vi "FlatToRichnixnet_grpc_SetPropertyRequest.vi"(5 "OutputClusterType":T1, 11 "InputCluster":T3) -> (3 "OutputCluster":T1)   [LabVIEW 2025, in "grpc-xnet_client.lvlib"]
uses:
  nixnet_grpc_SetPropertyRequest_Flat.ctl
  nidevice_grpc_Session_Flat.ctl
  nixnet_grpc_Property.ctl
  nixnet_grpc_U32Array_Flat.ctl
  nixnet_grpc_DbRefArray_Flat.ctl
  nixnet_grpc_EptRxFilterArray_Flat.ctl
  nixnet_grpc_EptRxFilter_Flat.ctl
  nixnet_grpc_SetPropertyRequest.ctl
  nixnet_grpc_SetPropertyRequest_property_id_enum/nixnet_grpc_SetPropertyRequest_property_id_enum.lvclass
  nixnet_grpc_SetPropertyRequest_property_value/nixnet_grpc_SetPropertyRequest_property_value.lvclass
  nidevice_grpc_Session.ctl
  grpc-xnet_client.lvlib
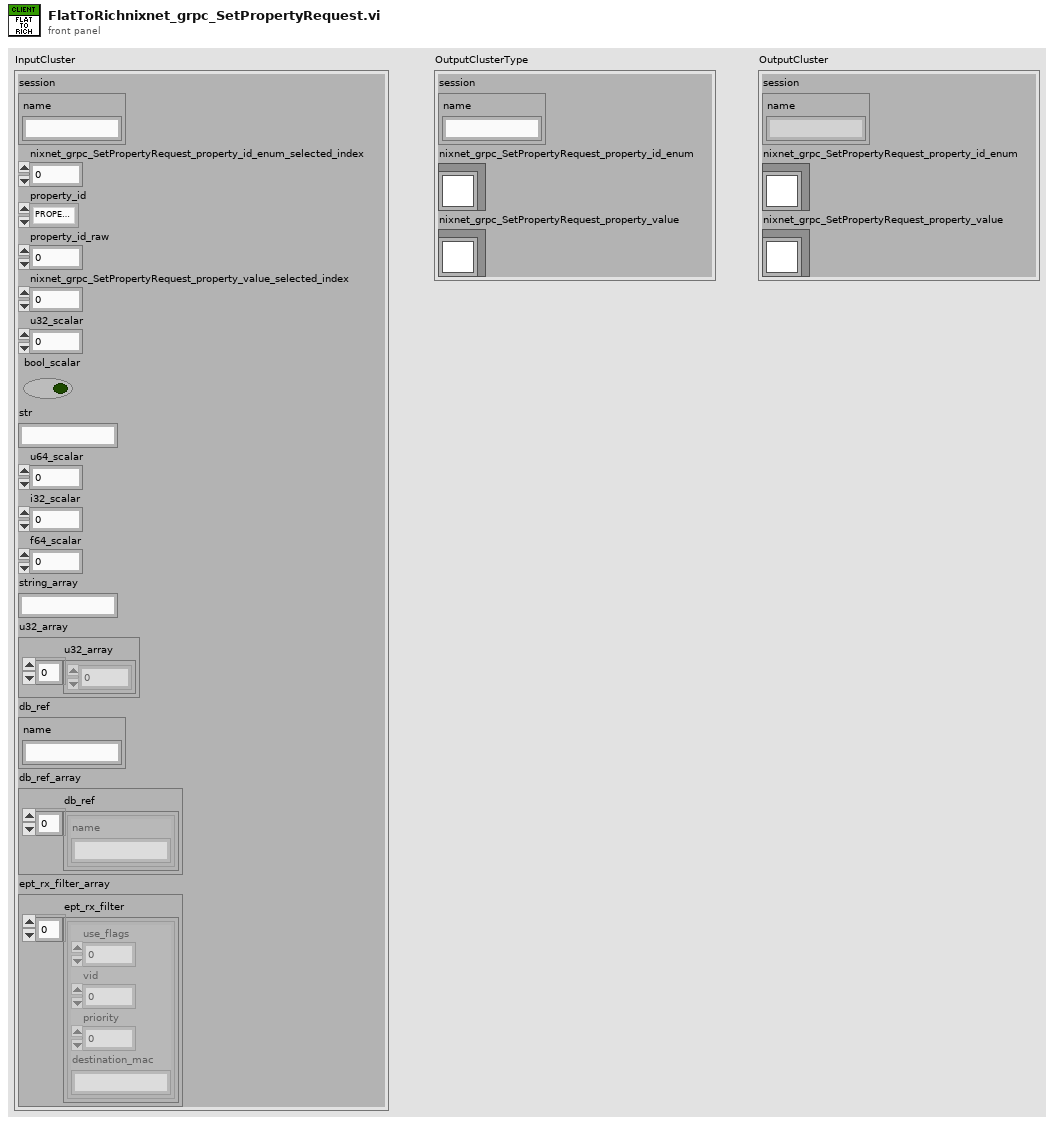
[diagram p1: front panel]
types:
  T1 = typedef "grpc-xnet_client.lvlib/nixnet_grpc_SetPropertyRequest.ctl" = cluster{"session":T2, "nixnet_grpc_SetPropertyRequest_property_id_enum":refnum<class "nixnet_grpc_SetPropertyRequest_property_id_enum.lvclass">, "nixnet_grpc_SetPropertyRequest_property_value":refnum<class "nixnet_grpc_SetPropertyRequest_property_value.lvclass">}
  T2 = typedef "grpc-xnet_client.lvlib/nidevice_grpc_Session.ctl" = cluster{"name":string}
  T3 = typedef "grpc-xnet_client.lvlib/nixnet_grpc_SetPropertyRequest_Flat.ctl" = cluster{"session":T4, "nixnet_grpc_SetPropertyRequest_property_id_enum_selected_index":i32, "property_id":T5, "property_id_raw":u32, "nixnet_grpc_SetPropertyRequest_property_value_selected_index":i32, "u32_scalar":u32, "bool_scalar":bool, "str":string, "u64_scalar":u64, "i32_scalar":i32, "f64_scalar":dbl, "string_array":string, "u32_array":T6, "db_ref":T4, "db_ref_array":T7, "ept_rx_filter_array":T8}
  T4 = typedef "grpc-xnet_client.lvlib/nidevice_grpc_Session_Flat.ctl" = cluster{"name":string}
  T5 = typedef "grpc-xnet_client.lvlib/nixnet_grpc_Property.ctl" = enum32{"PROPERTY_UNSPECIFIED", "PROPERTY_SESSION_APPLICATION_PROTOCOL", "PROPERTY_SESSION_AUTO_START", "PROPERTY_SESSION_CLUSTER_NAME", "PROPERTY_SESSION_DATABASE_NAME", "PROPERTY_SESSION_ENET_FRAME_FILTER", "PROPERTY_SESSION_ENET_LOG_ERROR", "PROPERTY_SESSION_ENET_LOG_FILE", "PROPERTY_SESSION_ENET_LOG_MODE", "PROPERTY_SESSION_ENET_LOG_ENABLE_MULTIPLE_FILES", "PROPERTY_SESSION_ENET_LOG_FILE_SIZE_THRESHOLD", "PROPERTY_SESSION_ENET_LOG_OPERATION", "PROPERTY_SESSION_ENET_NUM_FRAMES_RECEIVED", "PROPERTY_SESSION_ENET_SOURCE_MAC_ADDRESS_AUTO", "PROPERTY_SESSION_INTF_BAUD_RATE_64", "PROPERTY_SESSION_INTF_ADJUST_LOCAL_TIME", "PROPERTY_SESSION_INTF_BAUD_RATE", "PROPERTY_SESSION_INTF_BUS_ERR_TO_IN_STRM", "PROPERTY_SESSION_INTF_CAN_FD_BAUD_RATE_64", "PROPERTY_SESSION_INTF_CAN_DISABLE_PROT_EXCEPTION_HANDLING", "PROPERTY_SESSION_INTF_CAN_EDGE_FILTER", "PROPERTY_SESSION_INTF_CAN_EXT_TCVR_CONFIG", "PROPERTY_SESSION_INTF_CAN_FD_BAUD_RATE", "PROPERTY_SESSION_INTF_CAN_FD_ISO_MODE", "PROPERTY_SESSION_INTF_CAN_IO_MODE", "PROPERTY_SESSION_INTF_CAN_LSTN_ONLY", "PROPERTY_SESSION_INTF_CAN_PEND_TX_ORDER", "PROPERTY_SESSION_INTF_CAN_SING_SHOT", "PROPERTY_SESSION_INTF_CAN_TERM", "PROPERTY_SESSION_INTF_CAN_TCVR_STATE", "PROPERTY_SESSION_INTF_CAN_TCVR_TYPE", "PROPERTY_SESSION_INTF_CAN_TX_IO_MODE", "PROPERTY_SESSION_INTF_CAN_TRANSMIT_PAUSE", "PROPERTY_SESSION_INTF_ECHO_TX", "PROPERTY_SESSION_INTF_ENET_EPT_RECEIVE_FILTER", "PROPERTY_SESSION_INTF_ENET_EPT_TRANSMIT_BANDWIDTH", "PROPERTY_SESSION_INTF_ENET_IPV4_ADDRESS", "PROPERTY_SESSION_INTF_ENET_JUMBO_FRAMES", "PROPERTY_SESSION_INTF_ENET_LINK_SPEED", "PROPERTY_SESSION_INTF_ENET_LINK_SPEED_CONFIGURED", "PROPERTY_SESSION_INTF_ENET_MAC_ADDRESS", "PROPERTY_SESSION_INTF_ENET_OS_NETWORK_ADAPTER_DESCRIPTION", "PROPERTY_SESSION_INTF_ENET_OS_NETWORK_ADAPTER_NAME", "PROPERTY_SESSION_INTF_ENET_OPERATIONAL_STATUS", "PROPERTY_SESSION_INTF_ENET_OUT_STRM_TIMESCALE", "PROPERTY_SESSION_INTF_ENET_PHY_POWER_MODE", "PROPERTY_SESSION_INTF_ENET_PHY_STATE", "PROPERTY_SESSION_INTF_ENET_PORT_MODE", "PROPERTY_SESSION_INTF_ENET_SIGNAL_QUALITY", "PROPERTY_SESSION_INTF_ENET_SLEEP_CAPABILITY", "PROPERTY_SESSION_INTF_ENET_STATS_COUNTER_NAMES", "PROPERTY_SESSION_INTF_ENET_STATS_COUNTER_VALUES", "PROPERTY_SESSION_INTF_ENET_STATS_RX_BAD_FRAMES", "PROPERTY_SESSION_INTF_ENET_STATS_RX_BYTES", "PROPERTY_SESSION_INTF_ENET_STATS_RX_GOOD_FRAMES", "PROPERTY_SESSION_INTF_ENET_STATS_TX_BYTES", "PROPERTY_SESSION_INTF_ENET_STATS_TX_GOOD_FRAMES", "PROPERTY_SESSION_INTF_ENET_STATS_PHY_COUNTER_NAMES", "PROPERTY_SESSION_INTF_ENET_STATS_PHY_COUNTER_VALUES", "PROPERTY_SESSION_INTF_ENET_STATS_PHY_LOW_POWER_SLEEP", "PROPERTY_SESSION_INTF_ENET_STATS_PHY_SLEEP_FAILURE", "PROPERTY_SESSION_INTF_ENET_STATS_PHY_WAKEUP_FAILURE", "PROPERTY_SESSION_INTF_ENET_STATS_PHY_WAKEUP_PULSE", "PROPERTY_SESSION_INTF_ENET_STATS_PHY_WAKEUP_REQUEST", "PROPERTY_SESSION_INTF_ENET_TIME_ADJUST_NETWORK_TIME", "PROPERTY_SESSION_INTF_ENET_TIME_BMCA_ENABLED", "PROPERTY_SESSION_INTF_ENET_TIME_CLK_ACCURACY", "PROPERTY_SESSION_INTF_ENET_TIME_CLK_CLASS", "PROPERTY_SESSION_INTF_ENET_TIME_CLK_ID", "PROPERTY_SESSION_INTF_ENET_TIME_CLK_OFFSET_VAR", "PROPERTY_SESSION_INTF_ENET_TIME_GM_CLK_ACCURACY", "PROPERTY_SESSION_INTF_ENET_TIME_GM_CLK_CLASS", "PROPERTY_SESSION_INTF_ENET_TIME_GM_CLK_ID", "PROPERTY_SESSION_INTF_ENET_TIME_GM_CLK_OFFSET_VAR", "PROPERTY_SESSION_INTF_ENET_TIME_GM_PRIORITY_1", "PROPERTY_SESSION_INTF_ENET_TIME_GM_PRIORITY_2", "PROPERTY_SESSION_INTF_ENET_TIME_OFFSET_FROM_MASTER", "PROPERTY_SESSION_INTF_ENET_TIME_PORT_AS_CAPABLE", "PROPERTY_SESSION_INTF_ENET_TIME_PORT_ANNOUNCE_RECEIPT_TIMEOUT", "PROPERTY_SESSION_INTF_ENET_TIME_PORT_ANNOUNCE_TRANSMIT_ENABLED", "PROPERTY_SESSION_INTF_ENET_TIME_PORT_LOG_ANNOUNCE_INTERVAL", "PROPERTY_SESSION_INTF_ENET_TIME_PORT_LOG_ANNOUNCE_INTERVAL_CONFIGURED", "PROPERTY_SESSION_INTF_ENET_TIME_PORT_LOG_PDELAY_INTERVAL", "PROPERTY_SESSION_INTF_ENET_TIME_PORT_LOG_PDELAY_INTERVAL_CONFIGURED", "PROPERTY_SESSION_INTF_ENET_TIME_PORT_LOG_SYNC_INTERVAL", "PROPERTY_SESSION_INTF_ENET_TIME_PORT_LOG_SYNC_INTERVAL_CONFIGURED", "PROPERTY_SESSION_INTF_ENET_TIME_PORT_PDELAY_ENABLED", "PROPERTY_SESSION_INTF_ENET_TIME_PORT_STATE", "PROPERTY_SESSION_INTF_ENET_TIME_PORT_STATE_CONFIGURED", "PROPERTY_SESSION_INTF_ENET_TIME_PORT_PROP_DELAY", "PROPERTY_SESSION_INTF_ENET_TIME_PORT_PROP_DELAY_CONFIGURED", "PROPERTY_SESSION_INTF_ENET_TIME_PORT_PROP_DELAY_THRESHOLD", "PROPERTY_SESSION_INTF_ENET_TIME_PORT_STATS_COUNTER_NAMES", "PROPERTY_SESSION_INTF_ENET_TIME_PORT_STATS_COUNTER_VALUES", "PROPERTY_SESSION_INTF_ENET_TIME_PORT_STATS_RX_ANNOUNCE", "PROPERTY_SESSION_INTF_ENET_TIME_PORT_STATS_RX_PDELAY_REQUEST", "PROPERTY_SESSION_INTF_ENET_TIME_PORT_STATS_RX_SYNC", "PROPERTY_SESSION_INTF_ENET_TIME_PORT_STATS_TX_ANNOUNCE", "PROPERTY_SESSION_INTF_ENET_TIME_PORT_STATS_TX_PDELAY_REQUEST", "PROPERTY_SESSION_INTF_ENET_TIME_PORT_STATS_TX_SYNC", "PROPERTY_SESSION_INTF_ENET_TIME_PORT_SYNC_RECEIPT_TIMEOUT", "PROPERTY_SESSION_INTF_ENET_TIME_PORT_SYNC_STATUS", "PROPERTY_SESSION_INTF_ENET_TIME_PORT_SYNCED", "PROPERTY_SESSION_INTF_ENET_TIME_PRIORITY_1", "PROPERTY_SESSION_INTF_ENET_TIME_PRIORITY_2", "PROPERTY_SESSION_INTF_ENET_TIME_PROTOCOL", "PROPERTY_SESSION_INTF_ENET_TIME_PROTOCOL_ENABLED", "PROPERTY_SESSION_INTF_ENET_TIME_STEPS_TO_GM", "PROPERTY_SESSION_INTF_ENET_TRIGGER_PPS_SYNCED", "PROPERTY_SESSION_INTF_FLEX_RAY_ACC_START_RNG", "PROPERTY_SESSION_INTF_FLEX_RAY_ALW_HLT_CLK", "PROPERTY_SESSION_INTF_FLEX_RAY_ALW_PASS_ACT", "PROPERTY_SESSION_INTF_FLEX_RAY_AUTO_ASLP_WHN_STP", "PROPERTY_SESSION_INTF_FLEX_RAY_CLST_DRIFT_DMP", "PROPERTY_SESSION_INTF_FLEX_RAY_COLDSTART", "PROPERTY_SESSION_INTF_FLEX_RAY_CONNECTED_CHS", "PROPERTY_SESSION_INTF_FLEX_RAY_DEC_CORR", "PROPERTY_SESSION_INTF_FLEX_RAY_DELAY_COMP_A", "PROPERTY_SESSION_INTF_FLEX_RAY_DELAY_COMP_B", "PROPERTY_SESSION_INTF_FLEX_RAY_KEY_SLOT_ID", "PROPERTY_SESSION_INTF_FLEX_RAY_LATEST_TX", "PROPERTY_SESSION_INTF_FLEX_RAY_LIST_TIMO", "PROPERTY_SESSION_INTF_FLEX_RAY_MAC_INIT_OFF_A", "PROPERTY_SESSION_INTF_FLEX_RAY_MAC_INIT_OFF_B", "PROPERTY_SESSION_INTF_FLEX_RAY_MAX_DRIFT", "PROPERTY_SESSION_INTF_FLEX_RAY_MIC_INIT_OFF_A", "PROPERTY_SESSION_INTF_FLEX_RAY_MIC_INIT_OFF_B", "PROPERTY_SESSION_INTF_FLEX_RAY_MICROTICK", "PROPERTY_SESSION_INTF_FLEX_RAY_NULL_TO_IN_STRM", "PROPERTY_SESSION_INTF_FLEX_RAY_OFF_CORR", "PROPERTY_SESSION_INTF_FLEX_RAY_OFF_CORR_OUT", "PROPERTY_SESSION_INTF_FLEX_RAY_RATE_CORR", "PROPERTY_SESSION_INTF_FLEX_RAY_RATE_CORR_OUT", "PROPERTY_SESSION_INTF_FLEX_RAY_SAMP_PER_MICRO", "PROPERTY_SESSION_INTF_FLEX_RAY_SING_SLOT_EN", "PROPERTY_SESSION_INTF_FLEX_RAY_SLEEP", "PROPERTY_SESSION_INTF_FLEX_RAY_STATISTICS_EN", "PROPERTY_SESSION_INTF_FLEX_RAY_SYM_TO_IN_STRM", "PROPERTY_SESSION_INTF_FLEX_RAY_SYNC_STATUS", "PROPERTY_SESSION_INTF_FLEX_RAY_SYNC_CH_A_EVEN", "PROPERTY_SESSION_INTF_FLEX_RAY_SYNC_CH_A_ODD", "PROPERTY_SESSION_INTF_FLEX_RAY_SYNC_CH_B_EVEN", "PROPERTY_SESSION_INTF_FLEX_RAY_SYNC_CH_B_ODD", "PROPERTY_SESSION_INTF_FLEX_RAY_TERM", "PROPERTY_SESSION_INTF_FLEX_RAY_WAKEUP_CH", "PROPERTY_SESSION_INTF_FLEX_RAY_WAKEUP_PTRN", "PROPERTY_SESSION_INTF_NAME", "PROPERTY_SESSION_INTF_LIN_BREAK_DELIMITER_LENGTH", "PROPERTY_SESSION_INTF_LIN_BREAK_LENGTH", "PROPERTY_SESSION_INTF_LIN_CHECKSUM_TO_IN_STRM", "PROPERTY_SESSION_INTF_LIN_DIAG_P2_MIN", "PROPERTY_SESSION_INTF_LIN_DIAG_ST_MIN", "PROPERTY_SESSION_INTF_LIN_MASTER", "PROPERTY_SESSION_INTF_LIN_NO_RESPONSE_TO_IN_STRM", "PROPERTY_SESSION_INTF_LINO_STR_SLV_RSP_LST_BY_NAD", "PROPERTY_SESSION_INTF_LIN_SCHED_NAMES", "PROPERTY_SESSION_INTF_LIN_SLEEP", "PROPERTY_SESSION_INTF_LIN_ALW_START_WO_BUS_PWR", "PROPERTY_SESSION_INTF_LIN_TERM", "PROPERTY_SESSION_INTF_OUT_STRM_LIST", "PROPERTY_SESSION_INTF_OUT_STRM_LIST_BY_ID", "PROPERTY_SESSION_INTF_OUT_STRM_TIMNG", "PROPERTY_SESSION_INTF_SRC_TERM_START_TRIGGER", "PROPERTY_SESSION_INTF_START_TRIG_TO_IN_STRM", "PROPERTY_SESSION_LIST", "PROPERTY_SESSION_MODE", "PROPERTY_SESSION_NUM_IN_LIST", "PROPERTY_SESSION_NUM_FRAMES", "PROPERTY_SESSION_NUM_PEND", "PROPERTY_SESSION_NUM_UNUSED", "PROPERTY_SESSION_PAYLD_LEN_MAX", "PROPERTY_SESSION_PROTOCOL", "PROPERTY_SESSION_QUEUE_SIZE", "PROPERTY_SESSION_RESAMP_RATE", "PROPERTY_SESSION_J1939_ECU", "PROPERTY_SESSION_J1939_ECU_BUSY", "PROPERTY_SESSION_J1939_FILL_BYTE", "PROPERTY_SESSION_J1939_INCLUDE_DEST_ADDR_IN_PGN", "PROPERTY_SESSION_J1939_MAX_REPEAT_CTS", "PROPERTY_SESSION_J1939_ADDRESS", "PROPERTY_SESSION_J1939_NAME", "PROPERTY_SESSION_J1939_NUM_PACKETS_RECV", "PROPERTY_SESSION_J1939_NUM_PACKETS_RESP", "PROPERTY_SESSION_J1939_HOLD_TIME_TH", "PROPERTY_SESSION_J1939_RESPONSE_TIME_TR_GD", "PROPERTY_SESSION_J1939_RESPONSE_TIME_TR_SD", "PROPERTY_SESSION_J1939_TIMEOUT_T1", "PROPERTY_SESSION_J1939_TIMEOUT_T2", "PROPERTY_SESSION_J1939_TIMEOUT_T3", "PROPERTY_SESSION_J1939_TIMEOUT_T4", "PROPERTY_SESSION_J1939_WRITE_QUEUE_SIZE", "PROPERTY_SYS_CDAQ_PKT_TIME", "PROPERTY_SYS_DEV_REFS", "PROPERTY_SYS_INTF_REFS", "PROPERTY_SYS_INTF_REFS_ALL", "PROPERTY_SYS_INTF_REFS_CAN", "PROPERTY_SYS_INTF_REFS_ETHERNET", "PROPERTY_SYS_INTF_REFS_FLEX_RAY", "PROPERTY_SYS_INTF_REFS_LIN", "PROPERTY_SYS_VER_BUILD", "PROPERTY_SYS_VER_MAJOR", "PROPERTY_SYS_VER_MINOR", "PROPERTY_SYS_VER_PHASE", "PROPERTY_SYS_VER_UPDATE", "PROPERTY_DEV_FORM_FAC", "PROPERTY_DEV_INTF_REFS", "PROPERTY_DEV_INTF_REFS_ALL", "PROPERTY_DEV_NUM_PORTS", "PROPERTY_DEV_NUM_PORTS_ALL", "PROPERTY_DEV_NAME", "PROPERTY_DEV_PRODUCT_NUM", "PROPERTY_DEV_SER_NUM", "PROPERTY_DEV_SLOT_NUM", "PROPERTY_INTF_CAN_TERM_CAP", "PROPERTY_INTF_CAN_TCVR_CAP", "PROPERTY_INTF_DEV_REF", "PROPERTY_INTF_DONGLE_COMPATIBLE_FIRMWARE_VERSION", "PROPERTY_INTF_DONGLE_COMPATIBLE_REVISION", "PROPERTY_INTF_DONGLE_FIRMWARE_VERSION", "PROPERTY_INTF_DONGLE_ID", "PROPERTY_INTF_DONGLE_REVISION", "PROPERTY_INTF_DONGLE_STATE", "PROPERTY_INTF_NAME", "PROPERTY_INTF_NUM", "PROPERTY_INTF_PORT_NUM", "PROPERTY_INTF_PROTOCOL"}
  T6 = typedef "grpc-xnet_client.lvlib/nixnet_grpc_U32Array_Flat.ctl" = cluster{"u32_array":u32[]}
  T7 = typedef "grpc-xnet_client.lvlib/nixnet_grpc_DbRefArray_Flat.ctl" = cluster{"db_ref":T4[]}
  T8 = typedef "grpc-xnet_client.lvlib/nixnet_grpc_EptRxFilterArray_Flat.ctl" = cluster{"ept_rx_filter":T9[]}
  T9 = typedef "grpc-xnet_client.lvlib/nixnet_grpc_EptRxFilter_Flat.ctl" = cluster{"use_flags":u32, "vid":u32, "priority":u32, "destination_mac":string}
  T10 = typedef "grpc-xnet_client.lvlib/nixnet_grpc_U32Array.ctl" = cluster{"u32_array":u32[]}
  T11 = typedef "grpc-xnet_client.lvlib/nixnet_grpc_DbRefArray.ctl" = cluster{"db_ref":T2[]}
  T12 = typedef "grpc-xnet_client.lvlib/nixnet_grpc_EptRxFilterArray.ctl" = cluster{"ept_rx_filter":T13[]}
  T13 = typedef "grpc-xnet_client.lvlib/nixnet_grpc_EptRxFilter.ctl" = cluster{"use_flags":u32, "vid":u32, "priority":u32, "destination_mac":string}
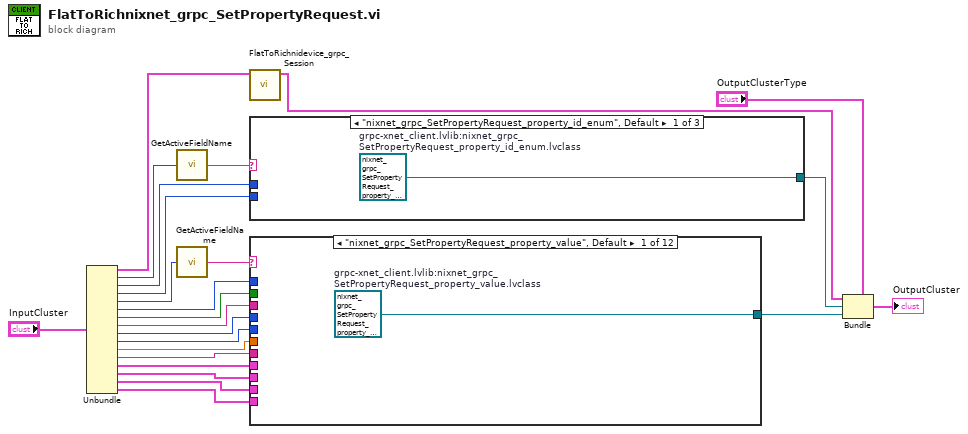
[diagram p0: block diagram]
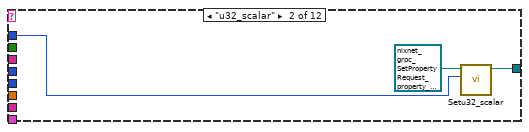
[diagram p2: hidden frame]
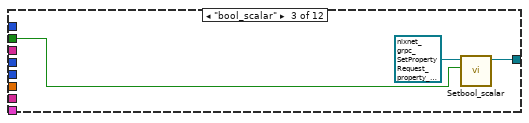
[diagram p3: hidden frame]
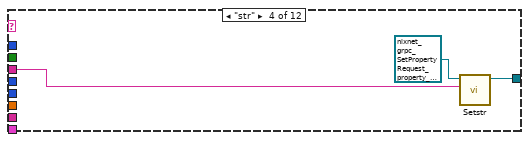
[diagram p4: hidden frame]
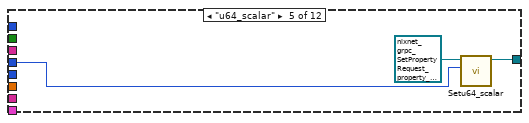
[diagram p5: hidden frame]
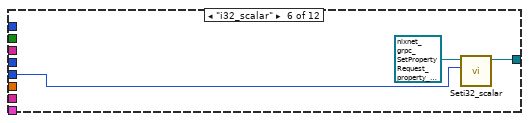
[diagram p6: hidden frame]
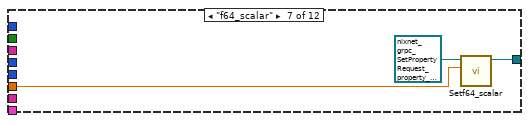
[diagram p7: hidden frame]
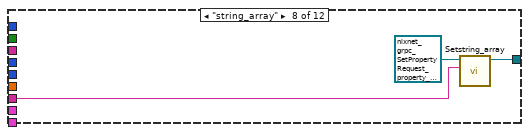
[diagram p8: hidden frame]
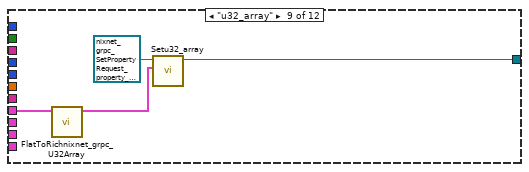
[diagram p9: hidden frame]
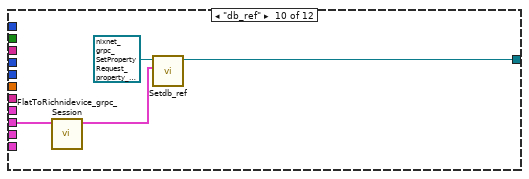
[diagram p10: hidden frame]
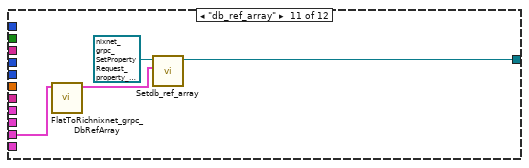
[diagram p11: hidden frame]
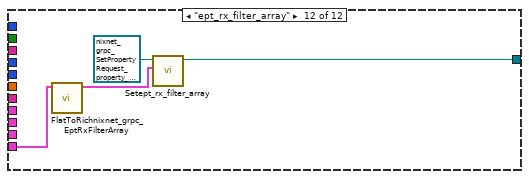
[diagram p12: hidden frame]
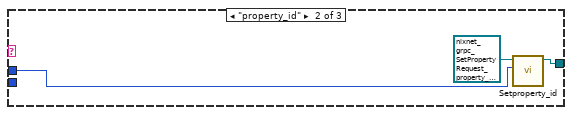
[diagram p13: hidden frame]
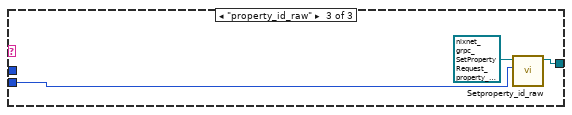
[diagram p14: hidden frame]
diagram:
  n1 = Unbundle "Unbundle"("InputCluster") -> ("session"=w21:T4, "nixnet_grpc_SetPropertyRequest_property_id_enum_selected_index"=w19:i32, "property_id"=w16:T5, "property_id_raw"=w15:u32, "nixnet_grpc_SetPropertyRequest_property_value_selected_index"=w14:i32, "u32_scalar"=w11:u32, "bool_scalar"=w10:bool, "str"=w9:string, "u64_scalar"=w8:u64, "i32_scalar"=w7:i32, "f64_scalar"=w6:dbl, "string_array"=w5:string, "u32_array"=w4:T6, "db_ref"=w3:T4, "db_ref_array"=w2:T7, "ept_rx_filter_array"=w1:T8)
  n2 = call "GetActiveFieldName.vi"("protobuf index"=w19) -> ("oneof field name"=w18:string)
  n3 = call "GetActiveFieldName.vi"("protobuf index"=w14) -> ("oneof field name"=w13:string)
  n4 = call "FlatToRichnidevice_grpc_Session.vi"("InputCluster"=w21) -> ("OutputCluster"=w20:T2)  [unwired: 10 in]
  n5 = case "nixnet_grpc_SetPropertyRequest_property_id_enum" shown="\"nixnet_grpc_SetPropertyRequest_property_id_enum\", Default" w18 {
    tunnel: [w25 w27 w30] -> w17
    tunnel: w16 -> [_ w28 _]
    tunnel: w15 -> [_ _ w31]
    frame "nixnet_grpc_SetPropertyRequest_property_id_enum", Default {
      w25 = refnum<class "nixnet_grpc_SetPropertyRequest_property_id_enum.lvclass"> refnum  # grpc-xnet_client.lvlib:nixnet_grpc_SetPropertyRequest_property_id_enum.lvclass
    }
    frame "property_id" {
      n6 = call "Setproperty_id.vi"("Set_Val"=w28, "OneOfTemplate in"=refnum<class "nixnet_grpc_SetPropertyRequest_property_id_enum.lvclass"> refnum) -> ("OneOfTemplate out"=w27:refnum<class "nixnet_grpc_SetPropertyRequest_property_id_enum.lvclass">)  [unwired: 8 in, 1 out]
    }
    frame "property_id_raw" {
      n7 = call "Setproperty_id_raw.vi"("Set_Val"=w31, "OneOfTemplate in"=refnum<class "nixnet_grpc_SetPropertyRequest_property_id_enum.lvclass"> refnum) -> ("OneOfTemplate out"=w30:refnum<class "nixnet_grpc_SetPropertyRequest_property_id_enum.lvclass">)  [unwired: 8 in, 1 out]
    }
  }
  n8 = case "nixnet_grpc_SetPropertyRequest_property_value" shown="\"nixnet_grpc_SetPropertyRequest_property_value\", Default" w13 {
    tunnel: [w32 w34 w37 w40 w43 w46 w49 w52 w55 w59 w63 w67] -> w12
    tunnel: w11 -> [_ w35 _ _ _ _ _ _ _ _ _ _]
    tunnel: w10 -> [_ _ w38 _ _ _ _ _ _ _ _ _]
    tunnel: w9 -> [_ _ _ w41 _ _ _ _ _ _ _ _]
    tunnel: w8 -> [_ _ _ _ w44 _ _ _ _ _ _ _]
    tunnel: w7 -> [_ _ _ _ _ w47 _ _ _ _ _ _]
    tunnel: w6 -> [_ _ _ _ _ _ w50 _ _ _ _ _]
    tunnel: w5 -> [_ _ _ _ _ _ _ w53 _ _ _ _]
    tunnel: w4 -> [_ _ _ _ _ _ _ _ w57 _ _ _]
    tunnel: w3 -> [_ _ _ _ _ _ _ _ _ w61 _ _]
    tunnel: w2 -> [_ _ _ _ _ _ _ _ _ _ w65 _]
    tunnel: w1 -> [_ _ _ _ _ _ _ _ _ _ _ w69]
    frame "nixnet_grpc_SetPropertyRequest_property_value", Default {
      w32 = refnum<class "nixnet_grpc_SetPropertyRequest_property_value.lvclass"> refnum  # grpc-xnet_client.lvlib:nixnet_grpc_SetPropertyRequest_property_value.lvclass
    }
    frame "u32_scalar" {
      n9 = call "Setu32_scalar.vi"("Set_Val"=w35, "OneOfTemplate in"=refnum<class "nixnet_grpc_SetPropertyRequest_property_value.lvclass"> refnum) -> ("OneOfTemplate out"=w34:refnum<class "nixnet_grpc_SetPropertyRequest_property_value.lvclass">)  [unwired: 8 in, 1 out]
    }
    frame "bool_scalar" {
      n10 = call "Setbool_scalar.vi"("Set_Val"=w38, "OneOfTemplate in"=refnum<class "nixnet_grpc_SetPropertyRequest_property_value.lvclass"> refnum) -> ("OneOfTemplate out"=w37:refnum<class "nixnet_grpc_SetPropertyRequest_property_value.lvclass">)  [unwired: 8 in, 1 out]
    }
    frame "str" {
      n11 = call "Setstr.vi"("Set_Val"=w41, "OneOfTemplate in"=refnum<class "nixnet_grpc_SetPropertyRequest_property_value.lvclass"> refnum) -> ("OneOfTemplate out"=w40:refnum<class "nixnet_grpc_SetPropertyRequest_property_value.lvclass">)  [unwired: 8 in, 1 out]
    }
    frame "u64_scalar" {
      n12 = call "Setu64_scalar.vi"("Set_Val"=w44, "OneOfTemplate in"=refnum<class "nixnet_grpc_SetPropertyRequest_property_value.lvclass"> refnum) -> ("OneOfTemplate out"=w43:refnum<class "nixnet_grpc_SetPropertyRequest_property_value.lvclass">)  [unwired: 8 in, 1 out]
    }
    frame "i32_scalar" {
      n13 = call "Seti32_scalar.vi"("Set_Val"=w47, "OneOfTemplate in"=refnum<class "nixnet_grpc_SetPropertyRequest_property_value.lvclass"> refnum) -> ("OneOfTemplate out"=w46:refnum<class "nixnet_grpc_SetPropertyRequest_property_value.lvclass">)  [unwired: 8 in, 1 out]
    }
    frame "f64_scalar" {
      n14 = call "Setf64_scalar.vi"("Set_Val"=w50, "OneOfTemplate in"=refnum<class "nixnet_grpc_SetPropertyRequest_property_value.lvclass"> refnum) -> ("OneOfTemplate out"=w49:refnum<class "nixnet_grpc_SetPropertyRequest_property_value.lvclass">)  [unwired: 8 in, 1 out]
    }
    frame "string_array" {
      n15 = call "Setstring_array.vi"("Set_Val"=w53, "OneOfTemplate in"=refnum<class "nixnet_grpc_SetPropertyRequest_property_value.lvclass"> refnum) -> ("OneOfTemplate out"=w52:refnum<class "nixnet_grpc_SetPropertyRequest_property_value.lvclass">)  [unwired: 8 in, 1 out]
    }
    frame "u32_array" {
      n16 = call "FlatToRichnixnet_grpc_U32Array.vi"("InputCluster"=w57) -> ("OutputCluster"=w56:T10)  [unwired: 10 in]
      n17 = call "Setu32_array.vi"("Set_Val"=w56, "OneOfTemplate in"=refnum<class "nixnet_grpc_SetPropertyRequest_property_value.lvclass"> refnum) -> ("OneOfTemplate out"=w55:refnum<class "nixnet_grpc_SetPropertyRequest_property_value.lvclass">)  [unwired: 8 in, 1 out]
    }
    frame "db_ref" {
      n18 = call "FlatToRichnidevice_grpc_Session.vi"("InputCluster"=w61) -> ("OutputCluster"=w60:T2)  [unwired: 10 in]
      n19 = call "Setdb_ref.vi"("Set_Val"=w60, "OneOfTemplate in"=refnum<class "nixnet_grpc_SetPropertyRequest_property_value.lvclass"> refnum) -> ("OneOfTemplate out"=w59:refnum<class "nixnet_grpc_SetPropertyRequest_property_value.lvclass">)  [unwired: 8 in, 1 out]
    }
    frame "db_ref_array" {
      n20 = call "FlatToRichnixnet_grpc_DbRefArray.vi"("InputCluster"=w65) -> ("OutputCluster"=w64:T11)  [unwired: 10 in]
      n21 = call "Setdb_ref_array.vi"("Set_Val"=w64, "OneOfTemplate in"=refnum<class "nixnet_grpc_SetPropertyRequest_property_value.lvclass"> refnum) -> ("OneOfTemplate out"=w63:refnum<class "nixnet_grpc_SetPropertyRequest_property_value.lvclass">)  [unwired: 8 in, 1 out]
    }
    frame "ept_rx_filter_array" {
      n22 = call "FlatToRichnixnet_grpc_EptRxFilterArray.vi"("InputCluster"=w69) -> ("OutputCluster"=w68:T12)  [unwired: 10 in]
      n23 = call "Setept_rx_filter_array.vi"("Set_Val"=w68, "OneOfTemplate in"=refnum<class "nixnet_grpc_SetPropertyRequest_property_value.lvclass"> refnum) -> ("OneOfTemplate out"=w67:refnum<class "nixnet_grpc_SetPropertyRequest_property_value.lvclass">)  [unwired: 8 in, 1 out]
    }
  }
  n24 = Bundle "Bundle"(cluster="OutputClusterType", "session"=w20, "nixnet_grpc_SetPropertyRequest_property_id_enum"=w17, "nixnet_grpc_SetPropertyRequest_property_value"=w12) -> (→"OutputCluster":T1)
